vi "binary_get_data.vi"(8 "error in":errorcluster, 10 "all in one package in":T1={"memory structure"={"length of metadata [byte]"=5, "length of page [byte]"=2048, "length of measurement data on page [byte]"=2028, "length of dataset [byte]"=6}, "actigraph settings"={"sampling frequency [Hz]"=0.0, "measurement interval [± g]"=0, "high precision?"=FALSE, "number of pages"=0, "rate code"=0, "range code"=0, "id"=0}, "time informations"={"starting time"=timestamp(0 s since 1904-01-01), "ending time"=timestamp(0 s since 1904-01-01), "dt[s]"=0.0, "sampling rate [Hz]"=0.0, "length"=0.0}, "measurement data"={"number of samples per axis"=0, "timestamp array"=[], "offset array"=[], "x, y, z axis data"=[], "normalised magnitude of acceleartion vectors"={"t0"=timestamp(0 s since 1904-01-01), "dt"=1.0, "Y"=[]}, "calibration coefficients"={"Sx"=0.0, "Ox"=0.0, "Sy"=0.0, "Oy"=0.0, "Sz"=0.0, "Oz"=0.0}, "statistics"={"mean of x axis acceleration"=0.0, "standard devation of x axis acceleration"=0.0, "mean of y axis acceleration"=0.0, "standard devation of y axis acceleration"=0.0, "mean of z axis acceleration"=0.0, "standard devation of z axis acceleration"=0.0, "mean of normalised magnitude of acceleration"=0.0, "standard devation of normalised magnitude of acceleration"=0.0}, "battery voltage"={"t0"=timestamp(0 s since 1904-01-01), "dt"=1.0, "Y"=[]}, "magnitude of acceleartion vectors"={"t0"=timestamp(0 s since 1904-01-01), "dt"=1.0, "Y"=[]}}} {"measurement data"."calibration coefficients"."Oz" format="%#_12g"; "measurement data"."calibration coefficients"."Sz" format="%#_12g"; "measurement data"."calibration coefficients"."Oy" format="%#_12g"; "measurement data"."calibration coefficients"."Sy" format="%#_12g"; "measurement data"."calibration coefficients"."Ox" format="%#_12g"; "measurement data"."calibration coefficients"."Sx" format="%#_12g"; "time informations"."length" format="%<%H:%M:%S%3u>t"; "actigraph settings"."id" format="%02d"; "actigraph settings"."range code" format="%02x"; "actigraph settings"."rate code" format="%02x"}, 11 "pages w/ first and last page":u8[](array[numeric])) -> (0 "error out":errorcluster, 3 "all in one package out":T1={"memory structure"={"length of metadata [byte]"=5, "length of page [byte]"=2048, "length of measurement data on page [byte]"=2028, "length of dataset [byte]"=6}, "actigraph settings"={"sampling frequency [Hz]"=0.0, "measurement interval [± g]"=0, "high precision?"=FALSE, "number of pages"=0, "rate code"=0, "range code"=0, "id"=0}, "time informations"={"starting time"=timestamp(0 s since 1904-01-01), "ending time"=timestamp(0 s since 1904-01-01), "dt[s]"=0.0, "sampling rate [Hz]"=0.0, "length"=0.0}, "measurement data"={"number of samples per axis"=0, "timestamp array"=[], "offset array"=[], "x, y, z axis data"=[], "normalised magnitude of acceleartion vectors"={"t0"=timestamp(0 s since 1904-01-01), "dt"=1.0, "Y"=[]}, "calibration coefficients"={"Sx"=0.0, "Ox"=0.0, "Sy"=0.0, "Oy"=0.0, "Sz"=0.0, "Oz"=0.0}, "statistics"={"mean of x axis acceleration"=0.0, "standard devation of x axis acceleration"=0.0, "mean of y axis acceleration"=0.0, "standard devation of y axis acceleration"=0.0, "mean of z axis acceleration"=0.0, "standard devation of z axis acceleration"=0.0, "mean of normalised magnitude of acceleration"=0.0, "standard devation of normalised magnitude of acceleration"=0.0}, "battery voltage"={"t0"=timestamp(0 s since 1904-01-01), "dt"=1.0, "Y"=[]}, "magnitude of acceleartion vectors"={"t0"=timestamp(0 s since 1904-01-01), "dt"=1.0, "Y"=[]}}} {"measurement data"."calibration coefficients"."Oz" format="%#_12g"; "measurement data"."calibration coefficients"."Sz" format="%#_12g"; "measurement data"."calibration coefficients"."Oy" format="%#_12g"; "measurement data"."calibration coefficients"."Sy" format="%#_12g"; "measurement data"."calibration coefficients"."Ox" format="%#_12g"; "measurement data"."calibration coefficients"."Sx" format="%#_12g"; "time informations"."length" format="%<%H:%M:%S%3u>t"; "actigraph settings"."id" format="%02d"; "actigraph settings"."range code" format="%02x"; "actigraph settings"."rate code" format="%02x"})   [LabVIEW 2020]
uses:
  Controls/control_all_in_one_package.ctl
  Controls/control_memory_structure.ctl
  Controls/control_measurement_settings.ctl
  Controls/control_time_informations.ctl
  Controls/control_measurement_data.ctl
  Controls/control_calibration_coefficients.ctl
  Controls/control_statistics.ctl
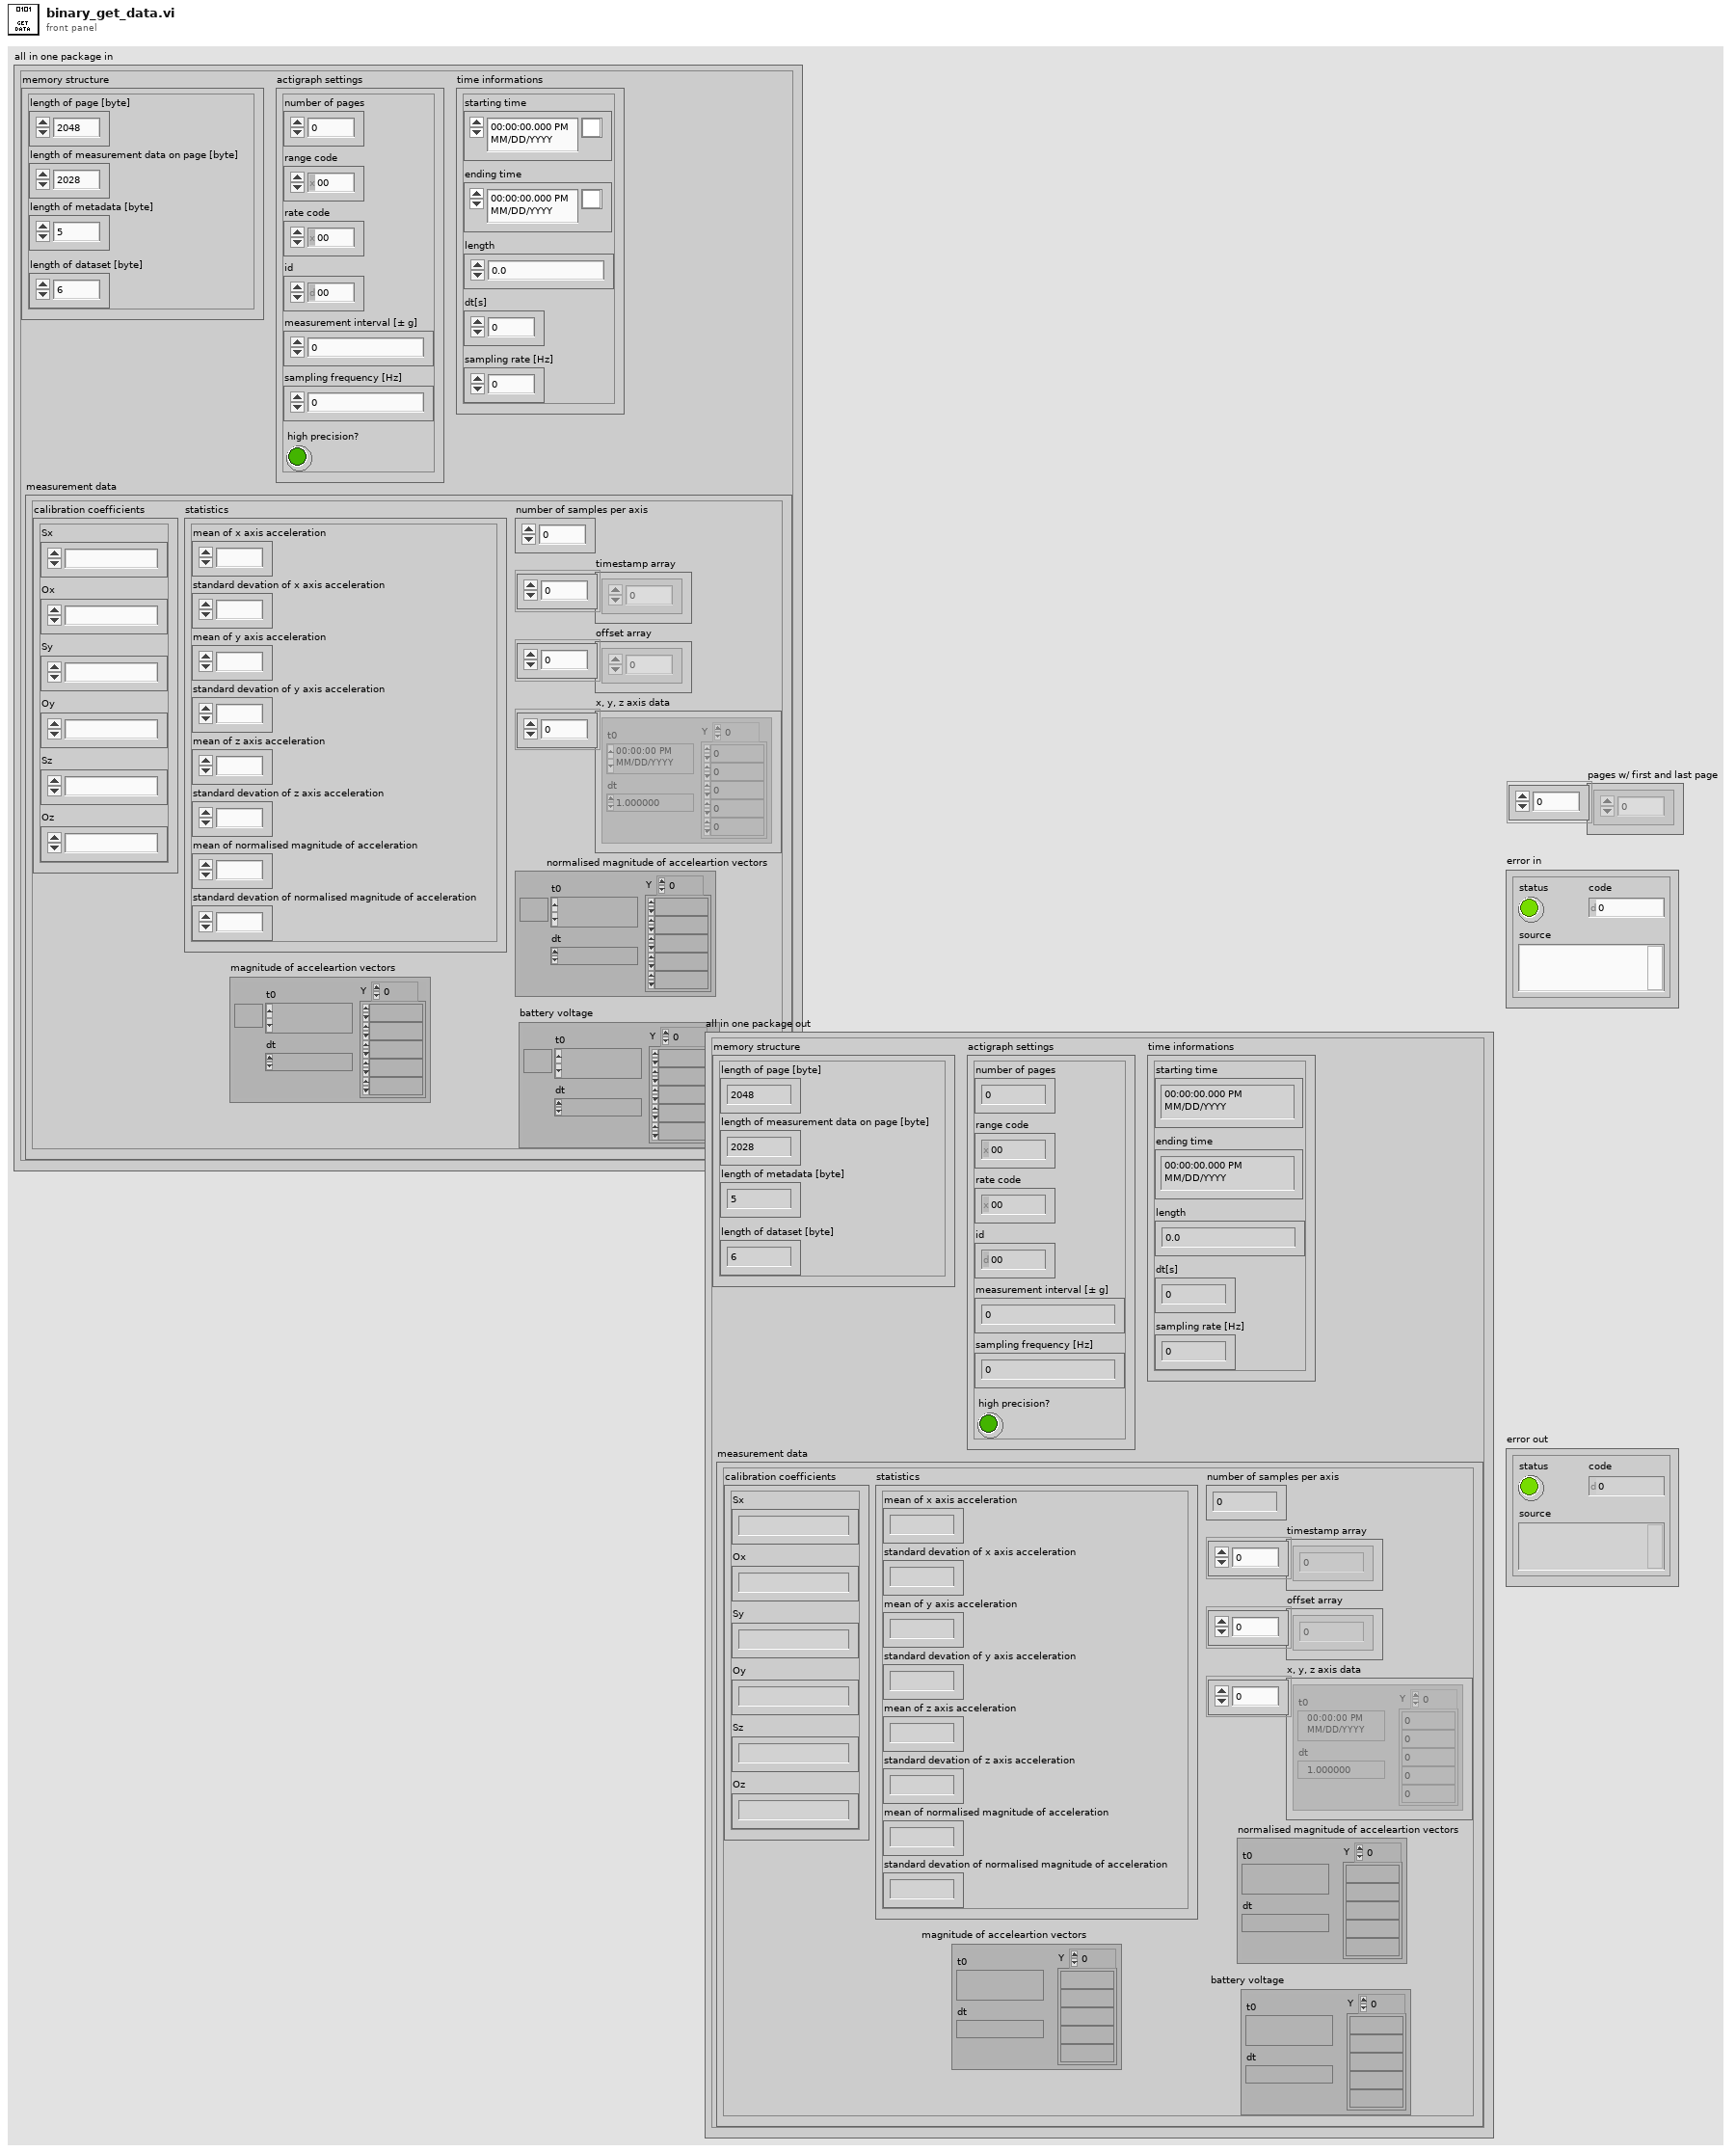
[diagram p1: front panel]
types:
  T1 = typedef "control_all_in_one_package.ctl" = cluster{"memory structure":T2, "actigraph settings":T3, "time informations":T4, "measurement data":T5}
  T2 = typedef "control_memory_structure.ctl" = cluster{"length of metadata [byte]":i32, "length of page [byte]":i32, "length of measurement data on page [byte]":i32, "length of dataset [byte]":i32}
  T3 = typedef "control_measurement_settings.ctl" = cluster{"sampling frequency [Hz]":dbl, "measurement interval [± g]":i32, "high precision?":bool, "number of pages":i32, "rate code":i32, "range code":i32, "id":i32}
  T4 = typedef "control_time_informations.ctl" = cluster{"starting time":timestamp, "ending time":timestamp, "dt[s]":dbl, "sampling rate [Hz]":dbl, "length":dbl}
  T5 = typedef "control_measurement_data.ctl" = cluster{"number of samples per axis":i32, "timestamp array":dbl[], "offset array":dbl[], "x, y, z axis data":waveform(dbl)[], "normalised magnitude of acceleartion vectors":waveform(dbl), "calibration coefficients":T6, "statistics":T7, "battery voltage":waveform(dbl), "magnitude of acceleartion vectors":waveform(dbl)}
  T6 = typedef "control_calibration_coefficients.ctl" = cluster{"Sx":dbl, "Ox":dbl, "Sy":dbl, "Oy":dbl, "Sz":dbl, "Oz":dbl}
  T7 = typedef "control_statistics.ctl" = cluster{"mean of x axis acceleration":dbl, "standard devation of x axis acceleration":dbl, "mean of y axis acceleration":dbl, "standard devation of y axis acceleration":dbl, "mean of z axis acceleration":dbl, "standard devation of z axis acceleration":dbl, "mean of normalised magnitude of acceleration":dbl, "standard devation of normalised magnitude of acceleration":dbl}
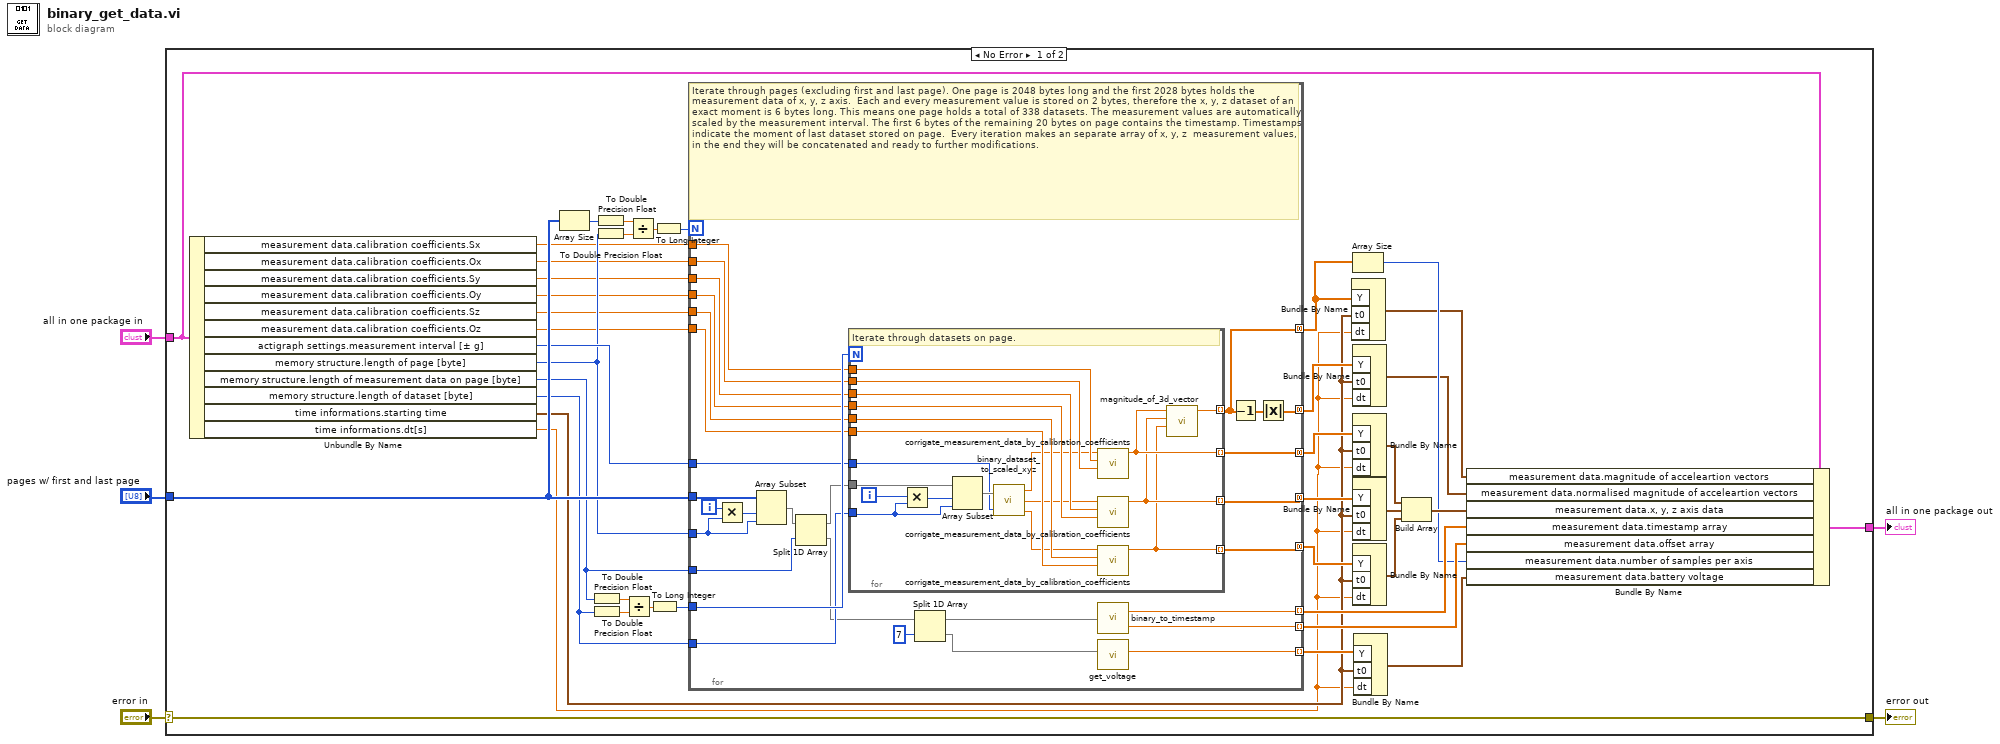
[diagram p0: block diagram]
diagram:
  n1 = case shown="No Error" "error in" {
    selector: "error in" -> [w46 w96]
    tunnel: "pages w/ first and last page" -> [w41 _]
    tunnel: [w46 w96] -> w4
    tunnel: "all in one package in" -> [w27 w95]
    tunnel: [w25 w95] -> w1
    frame No Error {
      n2 = Unbundle By Name(w27) -> ("measurement data.calibration coefficients.Sx"=w19:dbl, "measurement data.calibration coefficients.Ox"=w18:dbl, "measurement data.calibration coefficients.Sy"=w17:dbl, "measurement data.calibration coefficients.Oy"=w16:dbl, "measurement data.calibration coefficients.Sz"=w15:dbl, "measurement data.calibration coefficients.Oz"=w14:dbl, "actigraph settings.measurement interval [± g]"=w35:i32, "memory structure.length of page [byte]"=w34:i32, "memory structure.length of measurement data on page [byte]"=w33:i32, "memory structure.length of dataset [byte]"=w21:i32, "time informations.starting time"=w8:timestamp, "time informations.dt[s]"=w7:dbl)
      n3 = Array Size(array=w41) -> (size(s)=w45:i32)
      n4 = To Double Precision Float(number=w33) -> (double precision float=w37:dbl)
      n5 = To Double Precision Float(number=w21) -> (double precision float=w38:dbl)
      n6 = To Double Precision Float(number=w45) -> (double precision float=w42:dbl)
      n7 = To Double Precision Float(number=w34) -> (double precision float=w43:dbl)
      n8 = Divide(x=w37, y=w38) -> (x/y=w39:dbl)
      n9 = Divide(x=w42, y=w43) -> (x/y=w44:dbl)
      n10 = To Long Integer(number=w39) -> (32bit integer=w36:i32)
      n11 = To Long Integer(number=w44) -> (32bit integer=w40:i32)
      n12 = for {
        N: w40 -> [_]
        tunnel: [w62] -> w32 mode=concatenating
        tunnel: [w75] -> w31 mode=concatenating
        tunnel: [w74] -> w20 mode=concatenating
        tunnel: w33 -> [w70]
        tunnel: w41 -> [w72]
        tunnel: w34 -> [w67]
        tunnel: w36 -> [w71]
        tunnel: w21 -> [w66]
        tunnel: w35 -> [w65]
        tunnel: [w64] -> w24 mode=indexing
        tunnel: [w63] -> w23 mode=indexing
        tunnel: w19 -> [w56]
        tunnel: w18 -> [w57]
        tunnel: w17 -> [w58]
        tunnel: w16 -> [w59]
        tunnel: w15 -> [w60]
        tunnel: w14 -> [w61]
        tunnel: [w50] -> w12 mode=indexing
        tunnel: [w48] -> w11 mode=concatenating
        tunnel: [w47] -> w9 mode=concatenating
        i -> [w68]
        # "Iterate through pages (excluding first and last page). One page is 2048 bytes long and the first 2028 bytes holds the measurement data of x, y, z axis.  Each and every measurement value is stored on 2 bytes, therefore the x, y, z dataset of an exact moment is 6 bytes long. This means one page holds a total of 338 datasets. The measurement values are automatically scaled by the measurement interval. The first 6 bytes of the remaining 20 bytes on page contains the timestamp. Timestamps indicate the moment of last dataset stored on page.  Every iteration makes an separate array of x, y, z  measurement values, in the end they will be concatenated and ready to further modifications."
        n13 = Multiply(x=w68, y=w67) -> (x*y=w73:i32)
        n14 = Array Subset(array=w72, index=w73, length=w67) -> (w55:u8[])
        n15 = Split 1D Array(array=w55, index=w70) -> (first subarray=w69:u8[], second subarray=w54:u8[])
        n16 = for {
          N: w71 -> [_]
          tunnel: w69 -> [w94]
          tunnel: [w77] -> w75 mode=indexing
          tunnel: [w76] -> w74 mode=indexing
          tunnel: w66 -> [w90]
          tunnel: w65 -> [w89]
          tunnel: [w78] -> w62 mode=indexing
          tunnel: w61 -> [w83]
          tunnel: w60 -> [w84]
          tunnel: w59 -> [w85]
          tunnel: w58 -> [w86]
          tunnel: w57 -> [w87]
          tunnel: w56 -> [w88]
          tunnel: [w82] -> w47 mode=indexing
          i -> [w91]
          # "Iterate through datasets on page."
          n17 = Multiply(x=w91, y=w90) -> (x*y=w93:i32)
          n18 = Array Subset(array=w94, index=w93, length=w90) -> (w92:u8[])
          n19 = call "binary_dataset_to_scaled_xyz.vi"("binarySet"=w92, "measurementInterval"=w89) -> ("x axis value"=w81:dbl, "y axis value"=w80:dbl, "z axis value"=w79:dbl)
          n20 = call "corrigate_measurement_data_by_calibration_coefficients.vi"("Offset coeficient"=w87, "Scale coefficient"=w88, "Measurement value"=w81) -> ("Corrigated measurement value"=w78:dbl)  [unwired: 7 in, 1 out]
          n21 = call "corrigate_measurement_data_by_calibration_coefficients.vi"("Offset coeficient"=w85, "Scale coefficient"=w86, "Measurement value"=w80) -> ("Corrigated measurement value"=w77:dbl)  [unwired: 7 in, 1 out]
          n22 = call "corrigate_measurement_data_by_calibration_coefficients.vi"("Offset coeficient"=w83, "Scale coefficient"=w84, "Measurement value"=w79) -> ("Corrigated measurement value"=w76:dbl)  [unwired: 7 in, 1 out]
          n23 = call "magnitude_of_3d_vector.vi"("z axis component"=w76, "y axis component"=w77, "x axis component"=w78) -> ("magnitude of 3d vector"=w82:dbl)  [unwired: 7 in, 1 out]
        }
        n24 = Split 1D Array(array=w54, index=7) -> (first subarray=w52:u8[], second subarray=w51:u8[])
        n25 = call "binary_to_timestamp.vi"("binaryTimestampWithOffset"=w52) -> ("timestamp"=w64:dbl, "offset"=w63:dbl)
        n26 = call "get_voltage.vi"("Bytes of voltage"=w51) -> ("Voltage [V]"=w50:dbl)  [unwired: 9 in, 1 out]
        n27 = Decrement(x=w47) -> (x-1=w49:dbl[])
        n28 = Absolute Value(x=w49) -> (abs(x)=w48:dbl[])
      }
      n29 = Bundle By Name("Y"=w9, "t0"=w8, "dt"=w7) -> (w6:waveform(dbl))  [unwired: 1 in]
      n30 = Array Size(array=w9) -> (size(s)=w22:i32)
      n31 = Bundle By Name("Y"=w11, "t0"=w8, "dt"=w7) -> (w10:waveform(dbl))  [unwired: 1 in]
      n32 = Bundle By Name("Y"=w32, "t0"=w8, "dt"=w7) -> (w30:waveform(dbl))  [unwired: 1 in]
      n33 = Bundle By Name("Y"=w31, "t0"=w8, "dt"=w7) -> (w29:waveform(dbl))  [unwired: 1 in]
      n34 = Bundle By Name("Y"=w20, "t0"=w8, "dt"=w7) -> (w28:waveform(dbl))  [unwired: 1 in]
      n35 = Bundle By Name("Y"=w12, "t0"=w8, "dt"=w7) -> (w13:waveform(dbl))  [unwired: 1 in]
      n36 = Build Array(w30, w29, w28) -> (w26:waveform(dbl)[])
      n37 = Bundle By Name(cluster=w27, "measurement data.magnitude of acceleartion vectors"=w6, "measurement data.normalised magnitude of acceleartion vectors"=w10, "measurement data.x, y, z axis data"=w26, "measurement data.timestamp array"=w24, "measurement data.offset array"=w23, "measurement data.number of samples per axis"=w22, "measurement data.battery voltage"=w13) -> (w25:T1)
    }
    frame Error {
    }
  }
  "error out" <- w4
  "all in one package out" <- w1
